vi "x-axis.vi"(8 "error in (no error)":errorcluster, 11 "Magna Power Scan in":refnum<class "Magna Current Scan.lvclass">) -> (0 "error out":errorcluster, 1 "Label":string, 2 "Unit":string, 3 "Magna Power Scan out":refnum<class "Magna Current Scan.lvclass">)   [LabVIEW 2017, in "Magna Current Scan.lvclass"]
uses:
  Magna Current Scan.lvclass
  Scanner/Scanner.lvclass
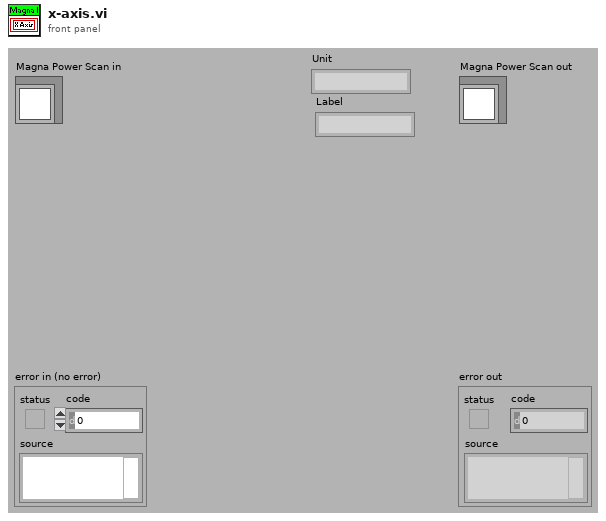
[diagram p1: front panel]
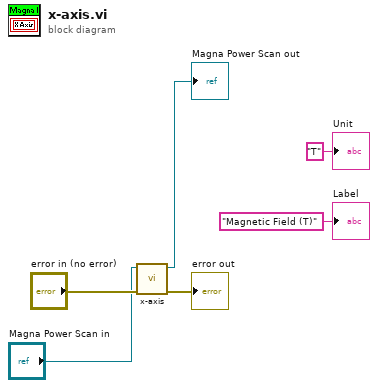
[diagram p0: block diagram]
diagram:
  n1 = call-parent "x-axis.vi"("error in (no error)"="error in (no error)", "Scanner in"="Magna Power Scan in") -> ("error out"=→"error out":errorcluster, "Scanner out"=→"Magna Power Scan out":refnum<class "Magna Current Scan.lvclass">)  [unwired: 6 in, 2 out]
  "Label" <- "Magnetic Field (T)" ("Label")
  "Unit" <- "T" ("Unit")
